vi "run.vi"(8 "error in (no error)":errorcluster, 11 "DL090202ScanHead in":refnum<class "ScanHeadDL090202.lvclass">) -> (0 "error out":errorcluster, 3 "DL090202ScanHead out":refnum<class "ScanHeadDL090202.lvclass">)   [LabVIEW 2010, in "ScanHeadDL090202.lvclass"]
uses:
  ScanHeadDL090202.lvclass
  main/labview_source/controls/undock_button.ctl
  internal_trigger_enum.ctl
  ScanHeadDL090202.lvclass/ScanHeadDL090202.ctl
  state_enum.ctl
  state_data_cluster.ctl
  GenericScanHead/GenericScanHead/GenericScanHead.lvclass
  Trajectory/GenericTrajectory/GenericTrajectory/GenericTrajectory.lvclass
  Trajectory/TrajectoryDL091126GenericVoxel/TrajectoryDL091126GenericVoxel/TrajectoryDL091126GenericVoxel.lvclass
  <vilib>/Utility/inputDevices.llb/closeKeyboard.vi
  <vilib>/Utility/inputDevices.llb/closeMouse.vi
  common/classes/ErrorController/ErrorController/class_data.vi
  <vilib>/Utility/inputDevices.llb/keyboardAcquire.vi
  <vilib>/Utility/inputDevices.llb/mouseAcquire.vi
  common/classes/ErrorController/ErrorController/ErrorController.lvclass
panel:
  in  "button:undock":T1
  in  "Tab Control":enum32{"user", "help", "debug", "about"}(tab)
  in  "zoom":dbl(slide)=1.0 min=1.0 max=20.0 step=0.1 scale=1.0..20.0
  in  "offset tabs":enum32{"fine", "coarse"}(tab)
  in  "x offset":dbl[unit](slide) scale format="%#_3g"
  in  "z offset":dbl[unit](slide)
  in  "y offset":dbl[unit](slide) scale format="%#_3g"
  in  "zero offset":bool
  in  "zero angles":bool
  in  "laser intensity (%)":dbl(slide)=14.5 caption="intensity (%)" min=0.001 max=100.0 step=0.1 scale=0.0..100.0
  in  "z angle":dbl[unit](slide) min=0.0 max=6.283185307179586 step=0.01745329238474369
  in  "x angle":dbl[unit](slide) caption="X amplitude" min=0.0 max=3.141592653589793 step=0.01745329238474369
  in  "misc tabs":enum32{"scanner-delay correction"}(tab)
  in  "x scanner":i32(slide) scale=-10.0..100.0
  in  "z scanner":i32(slide) scale=-10.0..100.0
  in  "y scanner":i32(slide) scale=-10.0..100.0
  in  "saveTrajectoryButton":bool
  out "state machine error":errorcluster
  in  "stop":bool
  out "statechart loop counter":i32
  out "evt lp error":errorcluster
  out "# elements in trigger queue":i32
  out "current action?":T2
  out "internal triggers":T2[](array[typedef])
  # "translation"
  # "rotation & tilting"
  # "Short-cuts\n\nLaser intensity: Mouse scroll wheel while space bar is pressed\n\nZoom: Mouse scroll wheel while Ctrl key is pressed\n\nToggling between horizontal and vertical plane imaging: press Ctrl-space"
  # "ScanHeadDL090202"
  # "Author: Dominik Langer, University of Zurich"
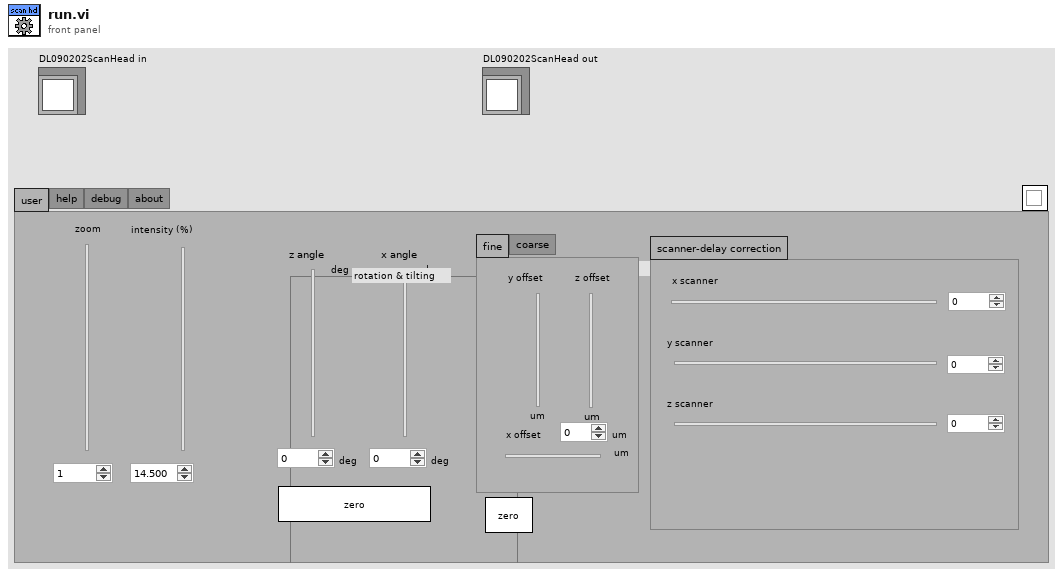
[diagram p1: front panel]
types:
  T1 = typedef "undock_button.ctl" = bool
  T2 = typedef "ScanHeadDL090202.lvclass/internal_trigger_enum.ctl" = enum16{"NULL", "initialise", "terminate", "start scanning", "stop scanning", "scale", "rotate", "tilt", "translate", "update modifiers", "fetch trajectory", "set run mode", "initialise scanners", "terminate scanners", "generate trajectory", "prepare writing", "write"}
  T3 = typedef "ScanHeadDL090202.lvclass/state_enum.ctl" = enum16{"idle", "initialising", "terminating", "writing"}
  T4 = typedef "ScanHeadDL090202.lvclass/state_data_cluster.ctl" = cluster{"already running?":bool, "new trajectory received?":bool, "fresh scan signals?":bool, "writing finished?":bool, "any trajectory received?":bool}
  T5 = enum16{"0", "1", "2", "3", "4", "5", "6", "7", "8", "9", "A", "B", "C", "D", "E", "F", "G", "H", "I", "J", "K", "L", "M", "N", "O", "P", "Q", "R", "S", "T", "U", "V", "W", "X", "Y", "Z", "F1", "F2", "F3", "F4", "F5", "F6", "F7", "F8", "F9", "F10", "F11", "F12", "F13", "F14", "F15", "ADD", "BACK", "BACKSLASH", "CAPITAL", "COMMA", "DECIMAL", "DELETE", "DIVIDE", "DOWN", "END", "EQUALS", "ESCAPE", "GRAVE (`)", "HOME", "INSERT", "LBRACKET", "LCONTROL", "LEFT", "L ALT", "LSHIFT", "LWIN", "MINUS", "MULTIPLY", "NEXT", "NUMLOCK", "NUMPAD_0", "NUMPAD_1", "NUMPAD_2", "NUMPAD_3", "NUMPAD_4", "NUMPAD_5", "NUMPAD_6", "NUMPAD_7", "NUMPAD_8", "NUMPAD_9", "PAUSE", "PERIOD", "PRIOR (PG UP)", "RBRACKET", "RCONTROL", "RETURN", "RIGHT", "R ALT", "RSHIFT", "RWIN", "SCROLL", "SEMICOLON", "SLASH", "SPACE", "SUBTRACT", "TAB", "UP", "ENTER (num pad)", "' (quote)"}
  T6 = typedef "main_trigger_enum.ctl" = enum16{"NULL", "initialise", "terminate", "start", "stop", "change objective", "change experimentController", "change imagingMode", "save notebook", "started saving", "finished saving", "expCtr ready", "expCtr missing", "imgMd ready", "imgMd missing", "scanHd ready", "scanHd missing", "DAQ ready", "DAQ missing", "imgAsm ready", "imgAsm missing", "dataColl ready", "dataColl missing", "display ready", "display missing", "analysr ready", "analysr missing", "instrmnt ready", "instrmnt missing", "stimltr ready", "stimltr missing", "stage ready", "stage missing"}
  T7 = enum16{"0", "1", "2", "3", "4", "5", "6", "7", "8", "9", "A", "B", "C", "D", "E", "F", "G", "H", "I", "J", "K", "L", "M", "N", "O", "P", "Q", "R", "S", "T", "U", "V", "W", "X", "Y", "Z", "F1", "F2", "F3", "F4", "F5", "F6", "F7", "F8", "F9", "F10", "F11", "F12", "F13", "F14", "F15", "ADD", "BACK", "BACKSLASH", "CAPITAL", "COMMA", "DECIMAL", "DELETE", "DIVIDE", "DOWN", "END", "EQUALS", "ESCAPE", "GRAVE (`)", "HOME", "INSERT", "LBRACKET", "LCONTROL", "LEFT", "L ALT", "LSHIFT", "LWIN", "MINUS", "MULTIPLY", "NEXT", "NUMLOCK", "NUMPAD_0", "NUMPAD_1", "NUMPAD_2", "NUMPAD_3", "NUMPAD_4", "NUMPAD_5", "NUMPAD_6", "NUMPAD_7", "NUMPAD_8", "NUMPAD_9", "PAUSE", "PERIOD", "PRIOR (PG UP)", "RBRACKET", "RCONTROL", "RETURN", "RIGHT", "R ALT", "RSHIFT", "RWIN", "SCROLL", "SEMICOLON", "SLASH", "SPACE", "SUBTRACT", "TAB", "UP", "ENTER (num pad)", "' (quote)"}[]
  T8 = cluster{"Horizontal":i32, "Vertical":i32, "Scrolling":i32}
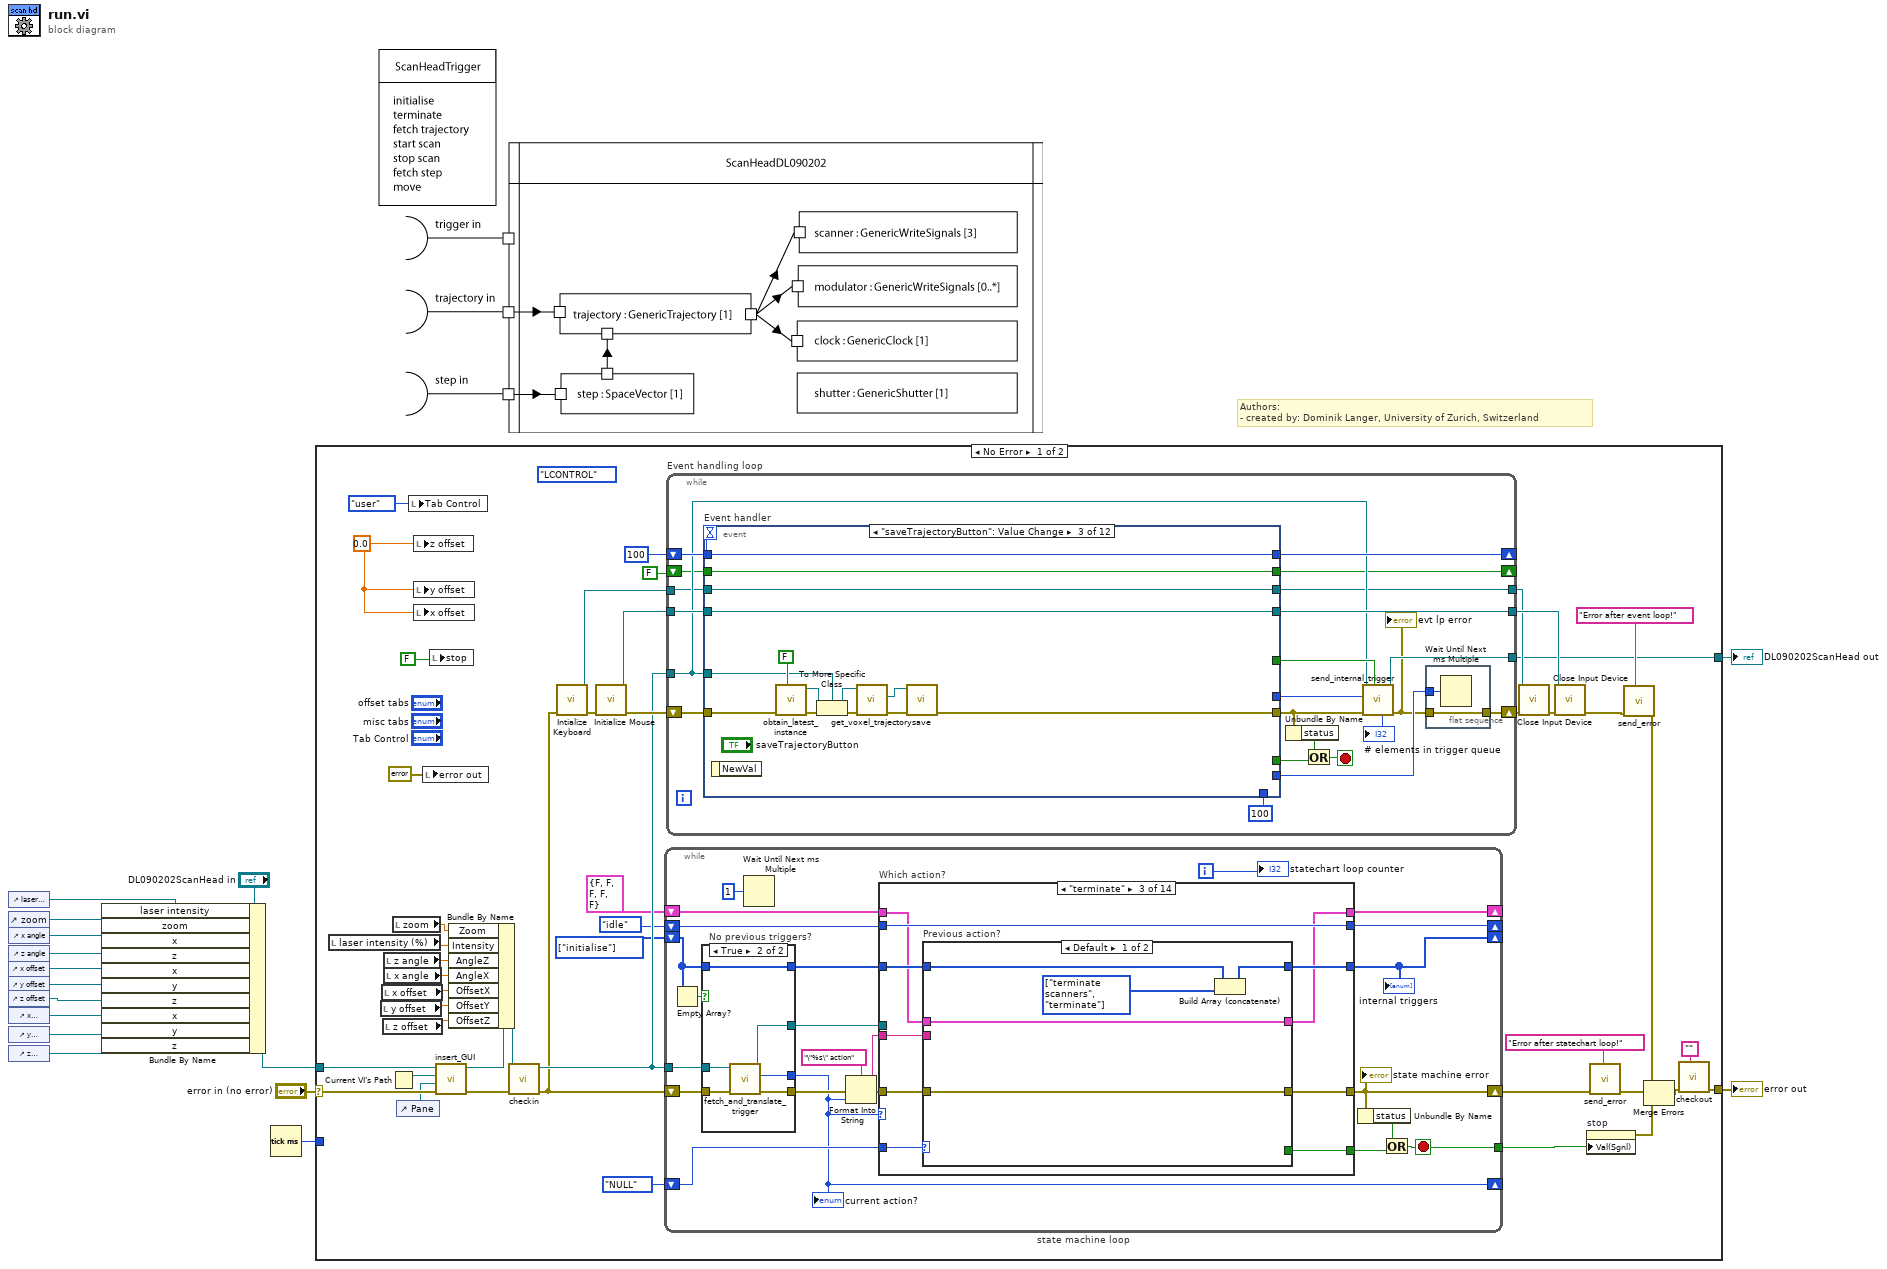
[diagram p0: block diagram]
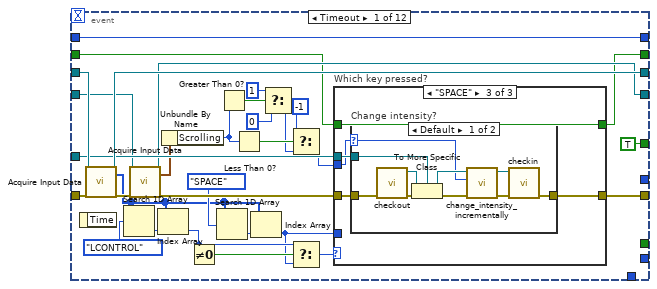
[diagram p2: hidden frame]
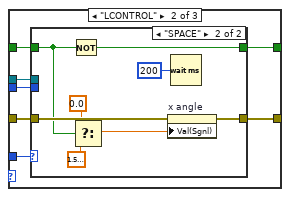
[diagram p4: hidden frame]
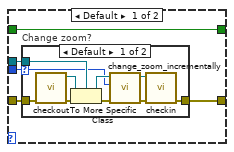
[diagram p5: hidden frame]
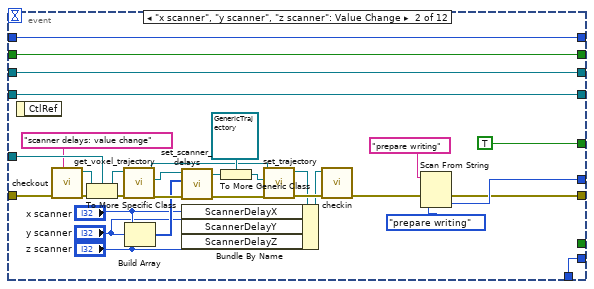
[diagram p8: hidden frame]
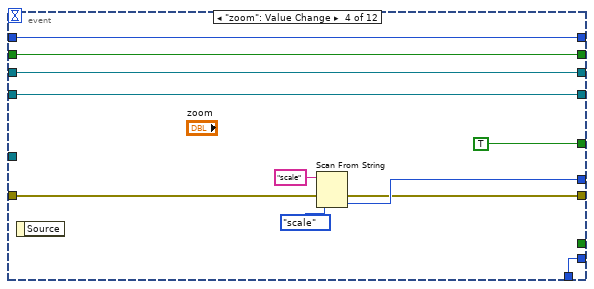
[diagram p9: hidden frame]
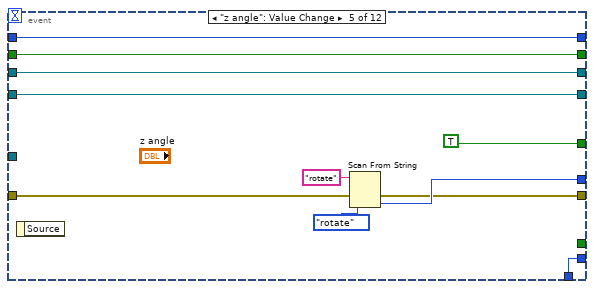
[diagram p10: hidden frame]
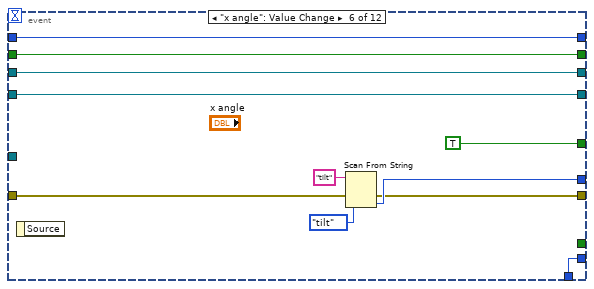
[diagram p11: hidden frame]
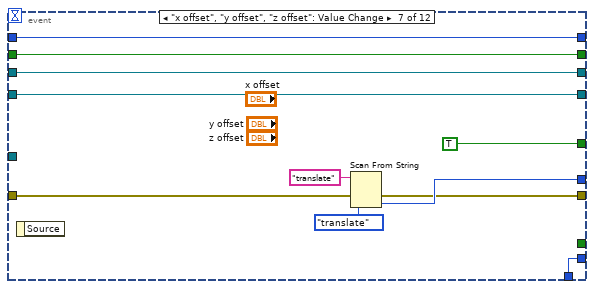
[diagram p12: hidden frame]
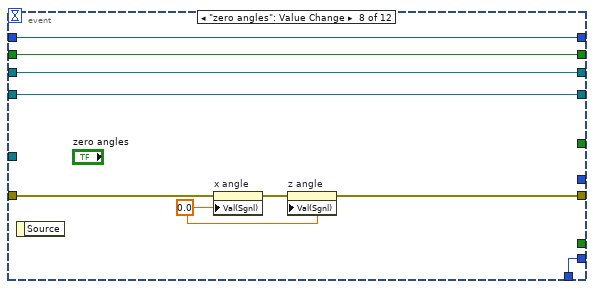
[diagram p13: hidden frame]
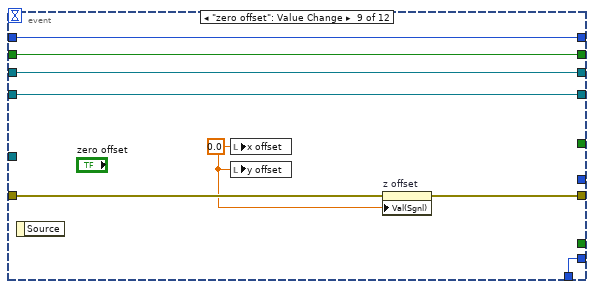
[diagram p14: hidden frame]
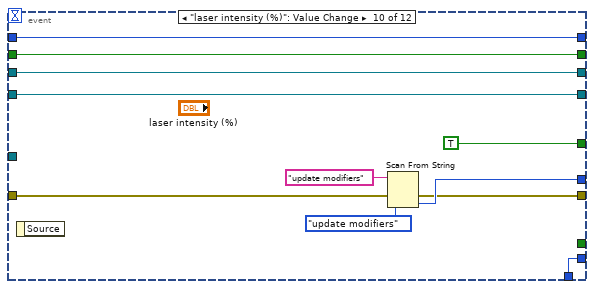
[diagram p15: hidden frame]
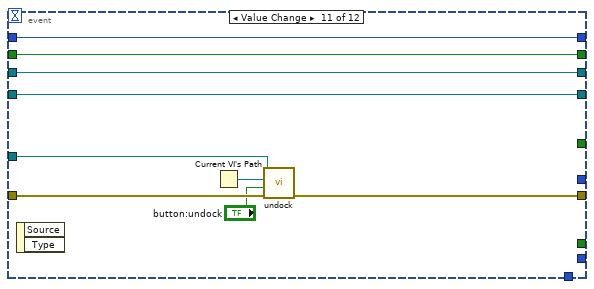
[diagram p16: hidden frame]
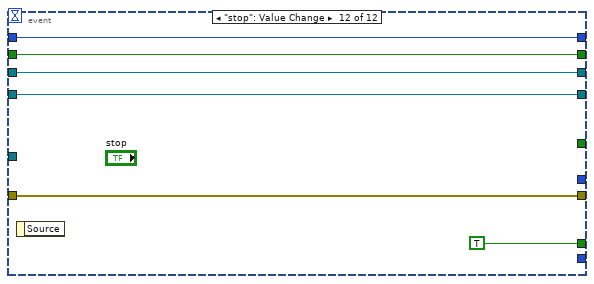
[diagram p17: hidden frame]
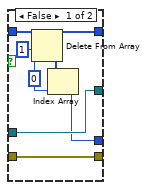
[diagram p18: hidden frame]
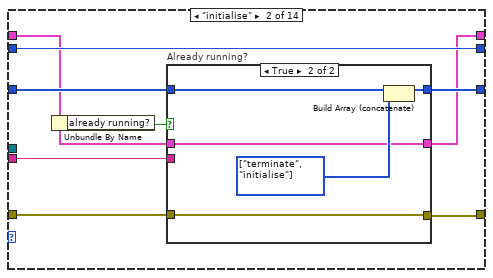
[diagram p20: hidden frame]
diagram:
  # "Authors: \n- created by: Dominik Langer, University of Zurich, Switzerland"
  n1 = control-ref of="laser intensity (%)"() -> (w9:refnum<vi>)
  n2 = control-ref of="zoom"() -> (w12:refnum<vi>)
  n3 = control-ref of="x angle"() -> (w10:refnum<vi>)
  n4 = control-ref of="z angle"() -> (w11:refnum<vi>)
  n5 = control-ref of="x offset"() -> (w6:refnum<vi>)
  n6 = control-ref of="y offset"() -> (w7:refnum<vi>)
  n7 = control-ref of="z offset"() -> (w8:refnum<vi>)
  n8 = control-ref of="x scanner"() -> (w3:refnum<vi>)
  n9 = control-ref of="y scanner"() -> (w4:refnum<vi>)
  n10 = control-ref of="z scanner"() -> (w2:refnum<vi>)
  n11 = Bundle By Name(cluster="DL090202ScanHead in", "laser intensity"=w9, "zoom"=w12, "x"=w10, "z"=w11, "x"=w6, "y"=w7, "z"=w8, "x"=w3, "y"=w4, "z"=w2) -> (w13:refnum<class "ScanHeadDL090202.lvclass">)
  n12 = Tick Count (ms)() -> (millisecond timer value=w1:u32)
  n13 = case shown="No Error" "error in (no error)" {
    selector: "error in (no error)" -> [w45 w583]
    tunnel: [w60 w583] -> w5
    tunnel: [w17 w582] -> w15
    tunnel: w13 -> [w44 w582]
    tunnel: w1 -> [_ _]
    frame No Error {
      (unwired) T5."LCONTROL" ("element")
      w25 = T2[] [enum."initialise"] items=["NULL", "initialise", "terminate", "start scanning", "stop scanning", "scale", "rotate", "tilt", "translate", "update modifiers", "fetch trajectory", "set run mode", "initialise scanners", "terminate scanners", "generate trajectory", "prepare writing", "write"]
      w55 = dbl[unit] 0.0 ("z offset")
      n14 = local read "laser intensity (%)"() -> (w52:dbl)
      n15 = local read "y offset"() -> (w47:dbl[unit])
      n16 = local read "x offset"() -> (w48:dbl[unit])
      n17 = local read "z offset"() -> (w46:dbl[unit])
      n18 = local read "z angle"() -> (w50:dbl[unit])
      n19 = local read "x angle"() -> (w49:dbl[unit])
      n20 = Current VI's Path() -> (path=w43:path)
      n21 = local read "zoom"() -> (w53:dbl)
      n22 = control-ref of="Pane"() -> (w42:refnum<vi>)
      n23 = local write "Tab Control"(enum32{"user", "help", "debug", "about"}."user" ("Tab Control")) -> ()
      n24 = local write "z offset"(w55) -> ()
      n25 = local write "y offset"(w55) -> ()
      n26 = local write "x offset"(w55) -> ()
      n27 = local write "error out"(errorcluster {"status"=FALSE, "code"=0, "source"=""} ("error out")) -> ()
      n28 = local write "stop"(FALSE) -> ()
      n29 = call-dynamic "insert_GUI.vi"("error in (no error)"=w45, "Pane"=w42, "VI path"=w43, "GenericComponent in"=w44) -> ("error out"=w28:errorcluster, "GenericComponent out"=w27:refnum<class "ScanHeadDL090202.lvclass">)  [unwired: 6 in]
      n30 = Bundle By Name(cluster=w27, "Zoom"=w53, "Intensity"=w52, "AngleZ"=w50, "AngleX"=w49, "OffsetX"=w48, "OffsetY"=w47, "OffsetZ"=w46) -> (w51:refnum<class "ScanHeadDL090202.lvclass">)
      n31 = call-dynamic "checkin.vi"("error in (no error)"=w28, "GenericScanHead in"=w51) -> ("error out"=w35:errorcluster, "GenericScanHead out"=w37:refnum<class "ScanHeadDL090202.lvclass">)  [unwired: 8 in]
      n32 = call <vilib>:"Intialize Keyboard.vi"("error in (no error)"=w35) -> ("error out"=w34:errorcluster, "device ID"=w33:refnum<k1>)  [unwired: 9 in]
      n33 = call <vilib>:"Initialize Mouse.vi"("error in (no error)"=w34) -> ("error out"=w54:errorcluster, "device ID"=w59:refnum<k1>)  [unwired: 9 in]
      n34 = while "state machine loop" {
        shift-right: [w306] -> _
        shift-left: T4 {"already running?"=FALSE, "new trajectory received?"=FALSE, "fresh scan signals?"=FALSE, "writing finished?"=FALSE, "any trajectory received?"=FALSE} -> [w307]
        tunnel: w37 -> [w321]
        shift-right: [w317] -> w23
        shift-left: w35 -> [w320]
        tunnel: [w319] -> w29
        shift-right: [w313] -> _
        shift-left: state_enum."idle" ("state") -> [w314]
        shift-right: [w312] -> _
        shift-left: w25 -> [w303]
        shift-right: [w300] -> _
        shift-left: internal_trigger_enum."NULL" ("internal trigger") -> [w305]
        i -> [w322]
        stop <- w319 stop-if-true
        n35 = Empty Array?(array=w303) -> (empty?=w304:bool)
        n36 = case "No previous triggers?" shown="True" w304 {
          tunnel: w321 -> [w328 w336]
          tunnel: w320 -> [w330 w335]
          tunnel: [w328 w334] -> w318
          tunnel: [w330 w333] -> w311
          tunnel: [w324 w332] -> w300
          tunnel: w303 -> [w329 w331]
          tunnel: [w327 w331] -> w302
          frame False {
            w325 = 0 ("index")
            n37 = Delete From Array(array=w329, length=1, index=w325) -> (deleted portion=w326:T2[], array with subset deleted=w327:T2[])
            n38 = Index Array(array=w326, index=w325) -> (element=w324:T2)
          }
          frame True {
            n39 = call-dynamic "fetch_and_translate_trigger.vi"("error in (no error)"=w335, "ScanHeadDL090202 in"=w336) -> ("error out"=w333:errorcluster, "internal trigger"=w332:T2, "ScanHeadDL090202 out"=w334:refnum<class "ScanHeadDL090202.lvclass">)  [unwired: 6 in, 1 out]
          }
        }
        "current action?" <- w300
        n40 = Wait Until Next ms Multiple(millisecond multiple=u32 1) -> ()  [unwired: 1 out]
        n41 = Format Into String(format string="\"%s\" action", error in=w311, w300) -> (resulting string=w308:string, error out=w310:errorcluster)  [unwired: 1 in]
        n42 = case "Which action?" shown="\"terminate\"" w300 {
          tunnel: w318 -> [_ _ _ w398 w412 _ _ _ w459 w474 w484 w518 w532 w553]
          tunnel: w310 -> [w338 w347 w376 w397 w411 w421 w432 w440 w453 w471 w486 w513 w530 w551]
          tunnel: [w338 w346 w375 w396 w410 w421 w432 w439 w454 w472 w485 w512 w529 w546] -> w317
          tunnel: [_ _ w368 _ _ _ _ _ _ _ _ _ _ _] -> w315
          tunnel: [w340 w349 w377 w407 w420 w422 w431 w446 w467 w482 w496 w522 w539 w558] -> w313
          tunnel: w314 -> [w340 w349 w377 w407 w420 w422 w431 w446 w467 w482 w496 w522 w539 w558]
          tunnel: w302 -> [w339 w345 w373 w406 w419 w425 w429 w438 w457 w470 w495 w511 w524 w545]
          tunnel: [w339 w344 w372 w406 w419 w424 w428 w437 w456 w469 w495 w510 w523 w545] -> w312
          tunnel: w308 -> [_ w348 w374 w399 w409 _ _ w441 w458 w473 w483 w517 w531 w552]
          tunnel: w307 -> [w337 w343 w370 w395 w408 w426 w430 w434 w466 w481 w494 w505 w528 w550]
          tunnel: [w337 w342 w369 w395 w408 w426 w430 w433 w466 w481 w494 w504 w527 w549] -> w306
          tunnel: w305 -> [_ _ w371 _ _ _ _ _ _ _ _ _ _ _]
          frame "NULL", Default {
          }
          frame "initialise" {
            n43 = Unbundle By Name(w343) -> ("already running?"=w341:bool)
            n44 = case "Already running?" shown="True" w341 {
              tunnel: w348 -> [w359 _]
              tunnel: w347 -> [w358 w367]
              tunnel: [w354 w367] -> w346
              tunnel: w345 -> [w353 w365]
              tunnel: [w353 w364] -> w344
              tunnel: w343 -> [w352 w363]
              tunnel: [w351 w363] -> w342
              frame False {
                n45 = call "checkout.vi"("locked by?"=w359, "error in (no error)"=w358) -> ("error out"=w357:errorcluster, "GenericScanHead out"=w360:refnum<class "GenericScanHead.lvclass">)  [unwired: 8 out]
                n46 = call-dynamic "construct.vi"("error in (no error)"=w357, "GenericPlugin in"=w360) -> ("error out"=w356:errorcluster, "GenericPlugin out"=w361:refnum<class "GenericScanHead.lvclass">)  [unwired: 2 in, 6 out]
                n47 = call-dynamic "initialise.vi"("error in (no error)"=w356, "GenericPlugin in"=w361) -> ("error out"=w355:errorcluster, "GenericPlugin out"=w362:refnum<class "GenericScanHead.lvclass">)  [unwired: 8 out]
                n48 = Bundle By Name(cluster=w352, "already running?"=TRUE) -> (w351:T4)
                n49 = call-dynamic "checkin.vi"("error in (no error)"=w355, "GenericScanHead in"=w362) -> ("error out"=w354:errorcluster)  [unwired: 8 in, 1 out]
              }
              frame True {
                w366 = T2[] [enum."terminate", enum."initialise"] items=["NULL", "initialise", "terminate", "start scanning", "stop scanning", "scale", "rotate", "tilt", "translate", "update modifiers", "fetch trajectory", "set run mode", "initialise scanners", "terminate scanners", "generate trajectory", "prepare writing", "write"]
                n50 = Build Array (concatenate)(w365, w366) -> (w364:T2[])
              }
            }
          }
          frame "terminate" {
            n51 = case "Previous action?" shown="Default" w371 {
              tunnel: w376 -> [w381 w390]
              tunnel: [w381 w389] -> w375
              tunnel: w374 -> [_ w388]
              tunnel: w373 -> [w379 w387]
              tunnel: [w382 w387] -> w372
              tunnel: [w380 w386] -> w369
              tunnel: w370 -> [w380 w385]
              tunnel: [_ TRUE] -> w368
              frame Default {
                w378 = T2[] [enum."terminate scanners", enum."terminate"] items=["NULL", "initialise", "terminate", "start scanning", "stop scanning", "scale", "rotate", "tilt", "translate", "update modifiers", "fetch trajectory", "set run mode", "initialise scanners", "terminate scanners", "generate trajectory", "prepare writing", "write"] ("array")
                n52 = Build Array (concatenate)(w379, w378) -> (w382:T2[])
              }
              frame "terminate scanners" {
                n53 = call "checkout.vi"("locked by?"=w388, "error in (no error)"=w390) -> ("error out"=w392:errorcluster, "GenericScanHead out"=w391:refnum<class "GenericScanHead.lvclass">)  [unwired: 8 out]
                n54 = call-dynamic "terminate.vi"("error in (no error)"=w392, "GenericPlugin in"=w391) -> ("error out"=w393:errorcluster, "GenericPlugin out"=w394:refnum<class "GenericScanHead.lvclass">)  [unwired: 8 out]
                n55 = Bundle By Name(cluster=w385, "already running?"=FALSE) -> (w386:T4)
                n56 = call-dynamic "checkin.vi"("error in (no error)"=w393, "GenericScanHead in"=w394) -> ("error out"=w389:errorcluster)  [unwired: 8 in, 1 out]
              }
            }
          }
          frame "start scanning" {
            n57 = call "checkout.vi"("locked by?"=w399, "error in (no error)"=w397) -> ("error out"=w405:errorcluster, "GenericScanHead out"=w404:refnum<class "GenericScanHead.lvclass">)  [unwired: 8 out]
            n58 = To More Specific Class(target class=w398, reference=w404, error in=w405) -> (specific class reference=w402:refnum<class "ScanHeadDL090202.lvclass">, error out=w403:errorcluster)
            n59 = call-dynamic "start.vi"("error in (no error)"=w403, "DL090202ScanHead in"=w402) -> ("error out"=w401:errorcluster, "DL090202ScanHead out"=w400:refnum<class "ScanHeadDL090202.lvclass">)  [unwired: 8 out]
            n60 = call-dynamic "checkin.vi"("error in (no error)"=w401, "GenericScanHead in"=w400) -> ("error out"=w396:errorcluster)  [unwired: 8 in, 1 out]
          }
          frame "stop scanning" {
            n61 = call "checkout.vi"("locked by?"=w409, "error in (no error)"=w411) -> ("error out"=w413:errorcluster, "GenericScanHead out"=w414:refnum<class "GenericScanHead.lvclass">)  [unwired: 8 out]
            n62 = To More Specific Class(target class=w412, reference=w414, error in=w413) -> (specific class reference=w416:refnum<class "ScanHeadDL090202.lvclass">, error out=w415:errorcluster)
            n63 = call-dynamic "stop.vi"("error in (no error)"=w415, "DL090202ScanHead in"=w416) -> ("error out"=w417:errorcluster, "DL090202ScanHead out"=w418:refnum<class "ScanHeadDL090202.lvclass">)  [unwired: 8 out]
            n64 = call-dynamic "checkin.vi"("error in (no error)"=w417, "GenericScanHead in"=w418) -> ("error out"=w410:errorcluster)  [unwired: 8 in, 1 out]
          }
          frame "scale".."tilt" {
            n65 = Build Array (concatenate)(w425, internal_trigger_enum."prepare writing" ("trigger")) -> (w424:T2[])
          }
          frame "translate", "update modifiers" {
            n66 = Build Array (concatenate)(w429, internal_trigger_enum."prepare writing" ("trigger")) -> (w428:T2[])
          }
          frame "fetch trajectory" {
            w435 = TRUE ("new trajectory received?")
            n67 = Unbundle By Name(w434) -> ("any trajectory received?"=w436:bool)
            n68 = call "checkout.vi"("locked by?"=w441, "error in (no error)"=w440) -> ("error out"=w442:errorcluster, "GenericScanHead out"=w443:refnum<class "GenericScanHead.lvclass">)  [unwired: 8 out]
            n69 = call-dynamic "fetch_trajectory.vi"("error in (no error)"=w442, "GenericScanHead in"=w443) -> ("error out"=w444:errorcluster, "GenericScanHead out"=w445:refnum<class "GenericScanHead.lvclass">)  [unwired: 8 out]
            n70 = call-dynamic "checkin.vi"("error in (no error)"=w444, "GenericScanHead in"=w445) -> ("error out"=w439:errorcluster)  [unwired: 8 in, 1 out]
            n71 = case "Any trajectory received?" shown="True" w436 {
              tunnel: w438 -> [w449 w451]
              tunnel: [w447 w450] -> w437
              frame False {
                n72 = Build Array (concatenate)(w449, internal_trigger_enum."generate trajectory" ("trigger")) -> (w447:T2[])
              }
              frame True {
                w452 = T2[] [enum."terminate scanners", enum."generate trajectory"] items=["NULL", "initialise", "terminate", "start scanning", "stop scanning", "scale", "rotate", "tilt", "translate", "update modifiers", "fetch trajectory", "set run mode", "initialise scanners", "terminate scanners", "generate trajectory", "prepare writing", "write"]
                n73 = Build Array (concatenate)(w451, w452) -> (w450:T2[])
              }
            }
            n74 = Bundle By Name(cluster=w434, "new trajectory received?"=w435, "any trajectory received?"=w435) -> (w433:T4)
          }
          frame "set run mode" {
            n75 = call "checkout.vi"("locked by?"=w458, "error in (no error)"=w453) -> ("error out"=w462:errorcluster, "GenericScanHead out"=w463:refnum<class "GenericScanHead.lvclass">)  [unwired: 8 out]
            n76 = To More Specific Class(target class=w459, reference=w463, error in=w462) -> (specific class reference=w464:refnum<class "ScanHeadDL090202.lvclass">, error out=w461:errorcluster)
            n77 = call-dynamic "update_run_mode.vi"("error in (no error)"=w461, "DL090202ScanHead in"=w464) -> ("error out"=w460:errorcluster, "DL090202ScanHead out"=w465:refnum<class "ScanHeadDL090202.lvclass">)  [unwired: 8 out]
            n78 = call-dynamic "checkin.vi"("error in (no error)"=w460, "GenericScanHead in"=w465) -> ("error out"=w454:errorcluster)  [unwired: 8 in, 1 out]
            n79 = Build Array (concatenate)(w457, internal_trigger_enum."prepare writing" ("trigger")) -> (w456:T2[])
          }
          frame "initialise scanners" {
            n80 = call "checkout.vi"("locked by?"=w473, "error in (no error)"=w471) -> ("error out"=w476:errorcluster, "GenericScanHead out"=w475:refnum<class "GenericScanHead.lvclass">)  [unwired: 8 out]
            n81 = To More Specific Class(target class=w474, reference=w475, error in=w476) -> (specific class reference=w478:refnum<class "ScanHeadDL090202.lvclass">, error out=w477:errorcluster)
            n82 = call-dynamic "initialise_scanners.vi"("error in (no error)"=w477, "DL090202ScanHead in"=w478) -> ("error out"=w479:errorcluster, "DL090202ScanHead out"=w480:refnum<class "ScanHeadDL090202.lvclass">)  [unwired: 8 out]
            n83 = call-dynamic "checkin.vi"("error in (no error)"=w479, "GenericScanHead in"=w480) -> ("error out"=w472:errorcluster)  [unwired: 8 in, 1 out]
            n84 = Build Array (concatenate)(w470, internal_trigger_enum."set run mode" ("trigger")) -> (w469:T2[])
          }
          frame "terminate scanners" {
            n85 = call "checkout.vi"("locked by?"=w483, "error in (no error)"=w486) -> ("error out"=w490:errorcluster, "GenericScanHead out"=w493:refnum<class "GenericScanHead.lvclass">)  [unwired: 8 out]
            n86 = To More Specific Class(target class=w484, reference=w493, error in=w490) -> (specific class reference=w492:refnum<class "ScanHeadDL090202.lvclass">, error out=w489:errorcluster)
            n87 = call-dynamic "terminate_scanners.vi"("error in (no error)"=w489, "DL090202ScanHead in"=w492) -> ("error out"=w488:errorcluster, "DL090202ScanHead out"=w491:refnum<class "ScanHeadDL090202.lvclass">)  [unwired: 8 out]
            n88 = call-dynamic "checkin.vi"("error in (no error)"=w488, "GenericScanHead in"=w491) -> ("error out"=w487:errorcluster)  [unwired: 8 in, 1 out]
            n89 = disable-structure shown="MAIN==1" {
              disable-tunnel: w487 -> [w499 w502]
              disable-tunnel: [w501 w502] -> w485
              frame condition #0 {
                n90 = call "string_to_main_trigger.vi"("error in (no error)"=w499, "trigger string"="scanHd missing") -> ("error out"=w498:errorcluster, "main trigger"=w500:T6)  [unwired: 8 in]
                n91 = call "send_main_trigger.vi"("error in (no error)"=w498, "trigger"=w500) -> ("error out"=w501:errorcluster)  [unwired: 9 in]
              }
              frame condition #1 (active) {
              }
            }
          }
          frame "generate trajectory" {
            n92 = call "checkout.vi"("locked by?"=w517, "error in (no error)"=w513) -> ("error out"=w516:errorcluster, "GenericScanHead out"=w520:refnum<class "GenericScanHead.lvclass">)  [unwired: 8 out]
            n93 = To More Specific Class(target class=w518, reference=w520, error in=w516) -> (specific class reference=w519:refnum<class "ScanHeadDL090202.lvclass">, error out=w515:errorcluster)
            n94 = Unbundle By Name(w505) -> ("new trajectory received?"=w508:bool)
            n95 = call-dynamic "generate_trajectory.vi"("error in (no error)"=w515, "DL090202ScanHead in"=w519) -> ("error out"=w514:errorcluster, "DL090202ScanHead out"=w521:refnum<class "ScanHeadDL090202.lvclass">)  [unwired: 8 out]
            n96 = call-dynamic "checkin.vi"("error in (no error)"=w514, "GenericScanHead in"=w521) -> ("error out"=w512:errorcluster)  [unwired: 8 in, 1 out]
            n97 = Bundle By Name(cluster=w505, "fresh scan signals?"=TRUE) -> (w504:T4)
            n98 = Select(t=internal_trigger_enum."initialise scanners" ("trigger"), s=w508, f=internal_trigger_enum."set run mode" ("trigger")) -> (s? t:f=w509:T2)
            n99 = Build Array (concatenate)(w511, w509) -> (w510:T2[])
          }
          frame "prepare writing" {
            n100 = call "checkout.vi"("locked by?"=w531, "error in (no error)"=w530) -> ("error out"=w537:errorcluster, "GenericScanHead out"=w538:refnum<class "GenericScanHead.lvclass">)  [unwired: 8 out]
            n101 = To More Specific Class(target class=w532, reference=w538, error in=w537) -> (specific class reference=w533:refnum<class "ScanHeadDL090202.lvclass">, error out=w536:errorcluster)
            n102 = call-dynamic "prepare_writing.vi"("error in (no error)"=w536, "DL090202ScanHead in"=w533) -> ("error out"=w535:errorcluster, "DL090202ScanHead out"=w534:refnum<class "ScanHeadDL090202.lvclass">)  [unwired: 1 in, 7 out]
            n103 = Build Array (concatenate)(w524, internal_trigger_enum."write" ("trigger")) -> (w523:T2[])
            n104 = call-dynamic "checkin.vi"("error in (no error)"=w535, "GenericScanHead in"=w534) -> ("error out"=w529:errorcluster)  [unwired: 8 in, 1 out]
            n105 = Bundle By Name(cluster=w528, "writing finished?"=FALSE) -> (w527:T4)
          }
          frame "write" {
            n106 = call "checkout.vi"("locked by?"=w552, "error in (no error)"=w551) -> ("error out"=w555:errorcluster, "GenericScanHead out"=w554:refnum<class "GenericScanHead.lvclass">)  [unwired: 8 out]
            n107 = To More Specific Class(target class=w553, reference=w554, error in=w555) -> (specific class reference=w557:refnum<class "ScanHeadDL090202.lvclass">, error out=w556:errorcluster)
            n108 = call-dynamic "write_signals.vi"("error in (no error)"=w556, "DL090202ScanHead in"=w557) -> ("error out"=w548:errorcluster, "finished?"=w544:bool, "DL090202ScanHead out"=w547:refnum<class "ScanHeadDL090202.lvclass">)  [unwired: 7 out]
            n109 = case "Writing finished?" shown="False" w544 {
              selector: w544 -> [_ w572]
              tunnel: w550 -> [w568 w575]
              tunnel: [w568 w574] -> w549
              tunnel: w548 -> [w562 w571]
              tunnel: w547 -> [w567 w570]
              tunnel: ["NULL" "scanHd ready"] -> w543
              tunnel: [w566 w571] -> w541
              tunnel: [w565 w570] -> w542
              frame False {
                n110 = Scan From String(input string="write", error in=w562, default 1=internal_trigger_enum."write" ("trigger")) -> (error out=w561:errorcluster, output 1=w563:T2)  [unwired: 2 in, 2 out]
                n111 = call-dynamic "send_internal_trigger.vi"("error in (no error)"=w561, "trigger"=w563, "DL090202ScanHead in"=w567) -> ("error out"=w566:errorcluster, "DL090202ScanHead out"=w565:refnum<class "ScanHeadDL090202.lvclass">)  [unwired: 1 in, 6 out]
              }
              frame True {
                w573 = FALSE
                n112 = Bundle By Name(cluster=w575, "new trajectory received?"=w573, "fresh scan signals?"=w573, "writing finished?"=w572) -> (w574:T4)
              }
            }
            n113 = call-dynamic "checkin.vi"("error in (no error)"=w541, "GenericScanHead in"=w542) -> ("error out"=w540:errorcluster)  [unwired: 8 in, 1 out]
            n114 = disable-structure shown="MAIN==1" {
              disable-tunnel: w540 -> [w577 w581]
              disable-tunnel: [w580 w581] -> w546
              disable-tunnel: w543 -> [w579 _]
              frame condition #0 {
                n115 = call "string_to_main_trigger.vi"("error in (no error)"=w577, "trigger string"=w579) -> ("error out"=w576:errorcluster, "main trigger"=w578:T6)  [unwired: 8 in]
                n116 = call "send_main_trigger.vi"("error in (no error)"=w576, "trigger"=w578) -> ("error out"=w580:errorcluster)  [unwired: 9 in]
              }
              frame condition #1 (active) {
              }
            }
          }
        }
        "state machine error" <- w317
        "internal triggers" <- w312
        n117 = Unbundle By Name(w317) -> ("status"=w316:bool)
        n118 = Or(x=w316, y=w315) -> (x .or. y?=w319:bool)
        "statechart loop counter" <- w322
      }
      n119 = while "Event handling loop" {
        shift-right: [w82] -> _
        shift-left: 100 -> [w83]
        tunnel: w37 -> [w77]
        tunnel: [w81] -> w17
        tunnel: w59 -> [w79]
        tunnel: [w78] -> w58
        tunnel: w33 -> [w72]
        tunnel: [w71] -> w32
        shift-right: [w65] -> w31
        shift-left: w54 -> [w84]
        shift-right: [w67] -> _
        shift-left: FALSE -> [w68]
        stop <- w74 stop-if-true
        n120 = event "Event handler" shown="[2] \"saveTrajectoryButton\": Value Change" {
          selector: _ -> [_ _ _ _ _ _ _ _ _ _ _ _]
          dyn-events: _ -> [_ _ _ _ _ _ _ _ _ _ _ _]
          timeout: w83 -> [_ _ _ _ _ _ _ _ _ _ _ _]
          tunnel: w84 -> [w115 w194 w209 w216 w226 w238 w248 w264 w272 w277 w289 w299]
          tunnel: [w111 w170 w201 w215 w227 w237 w249 w262 w271 w276 w288 w299] -> w76
          tunnel: [w117 w198 w212 w223 w234 w245 w256 w265 w273 w284 w293 w298] -> w82
          tunnel: w83 -> [w117 w198 w212 w223 w234 w245 w256 w265 w273 w284 w293 w298]
          tunnel: [_ _ _ _ _ _ _ _ _ _ _ TRUE] -> w73
          tunnel: [TRUE TRUE _ TRUE TRUE TRUE TRUE _ _ TRUE _ _] -> w80
          tunnel: w77 -> [w110 w195 w208 _ _ _ _ _ _ _ w290 _]
          tunnel: [_ w173 _ w217 w228 w239 w250 _ _ w279 _ _] -> w69
          tunnel: w79 -> [w106 w197 w211 w221 w232 w243 w254 w260 w269 w282 w292 w296]
          tunnel: [w105 w197 w211 w221 w232 w243 w254 w260 w269 w282 w292 w296] -> w78
          tunnel: w72 -> [w116 w169 w200 w220 w231 w242 w253 w259 w268 w281 w291 w295]
          tunnel: [w113 w169 w200 w220 w231 w242 w253 w259 w268 w281 w291 w295] -> w71
          tunnel: w68 -> [w88 w168 w199 w214 w225 w236 w247 w258 w267 w275 w285 w294]
          tunnel: [w87 w168 w199 w214 w225 w236 w247 w258 w267 w275 w285 w294] -> w67
          tunnel: [_ w167 _ w213 w224 w235 w246 w257 w266 w274 _ _] -> w66
          tunnel: u32 100 ("millisecond multiple") -> [_ w167 _ w213 w224 w235 w246 w257 w266 w274 _ _]
          event Timeout {
            n121 = event-data() -> ()  [unwired: 2 out]
            n122 = call-poly <vilib>:"Acquire Input Data.vi"("device ID"=w116, "error in (no error)"=w115) -> ("device ID"=w113:refnum<k1>, "keys pressed"=w102:T7, "error out"=w108:errorcluster)  [unwired: 15 in]
            n123 = Search 1D Array(1D array=w102, element=T5."LCONTROL") -> (index of element=w109:i32)  [unwired: 1 in]
            n124 = call-poly <vilib>:"Acquire Input Data.vi"("device ID"=w106, "error in (no error)"=w108) -> ("device ID"=w105:refnum<k1>, "axis info"=w104:T8, "error out"=w107:errorcluster)  [unwired: 14 in, 1 out]
            n125 = Index Array(array=w102, index=w109) -> (element=w100:T5)
            n126 = Unbundle By Name(w104) -> ("Scrolling"=w92:i32)
            n127 = Not Equal To 0?(x=w100) -> (x != 0?=w99:bool)
            n128 = Search 1D Array(1D array=w102, element=T5."SPACE") -> (index of element=w101:i32)  [unwired: 1 in]
            n129 = Greater Than 0?(x=w92) -> (x > 0?=w97:bool)
            n130 = Less Than 0?(x=w92) -> (x < 0?=w95:bool)
            n131 = Index Array(array=w102, index=w101) -> (element=w89:T5)
            n132 = Select(t=1, s=w97, f=0) -> (s? t:f=w93:i32)
            n133 = Select(t=-1, s=w95, f=w93) -> (s? t:f=w91:i32)
            n134 = Select(t=w100, s=w99, f=w89) -> (s? t:f=w98:T5)
            n135 = case "Which key pressed?" shown="\"SPACE\"" w98 {
              tunnel: w107 -> [w119 w125 w154]
              tunnel: [w119 w126 w153] -> w111
              tunnel: w110 -> [_ w124 w155]
              tunnel: w91 -> [_ w123 w152]
              tunnel: w89 -> [_ w122 _]
              tunnel: w88 -> [w118 w121 w151]
              tunnel: [w118 w120 w151] -> w87
              frame Default {
              }
              frame "LCONTROL" {
                n136 = case shown="\"SPACE\"" w122 {
                  tunnel: [w131 w149] -> w126
                  tunnel: w125 -> [w130 w150]
                  tunnel: w124 -> [w129 _]
                  tunnel: w123 -> [w128 _]
                  tunnel: w121 -> [w127 w144]
                  tunnel: [w127 w148] -> w120
                  frame Default {
                    n137 = case "Change zoom?" shown="Default" w128 {
                      selector: w128 -> [w132 _]
                      tunnel: w130 -> [w138 w142]
                      tunnel: [w140 w142] -> w131
                      tunnel: w129 -> [w134 _]
                      frame Default {
                        n138 = call "checkout.vi"("error in (no error)"=w138) -> ("error out"=w137:errorcluster, "GenericScanHead out"=w135:refnum<class "GenericScanHead.lvclass">)  [unwired: 9 in]
                        n139 = To More Specific Class(target class=w134, reference=w135, error in=w137) -> (specific class reference=w133:refnum<class "ScanHeadDL090202.lvclass">, error out=w136:errorcluster)
                        n140 = call "change_zoom_incrementally.vi"("error in (no error)"=w136, "mode"=w132, "ScanHeadDL090202 in"=w133) -> ("error out"=w141:errorcluster, "ScanHeadDL090202 out"=w139:refnum<class "ScanHeadDL090202.lvclass">)  [unwired: 7 in]
                        n141 = call-dynamic "checkin.vi"("error in (no error)"=w141, "GenericScanHead in"=w139) -> ("error out"=w140:errorcluster)  [unwired: 8 in, 1 out]
                      }
                      frame 0 {
                      }
                    }
                  }
                  frame "SPACE" {
                    n142 = Not(x=w144) -> (.not. x?=w148:bool)
                    n143 = Select(t=dbl[unit] 0.0 ("Value (Signaling)"), s=w144, f=dbl[unit] 1.5707963267948966) -> (s? t:f=w146:dbl[unit])
                    n144 = property on="x angle" class="Slide (strict)"(error in=w150, "Val(Sgnl)"=w146) -> (error out=w149:errorcluster)  [unwired: 1 in, 1 out]
                    n145 = Wait (ms)(milliseconds to wait=u32 200) -> ()  [unwired: 1 out]
                  }
                }
              }
              frame "SPACE" {
                n146 = case "Change intensity?" shown="Default" w152 {
                  selector: w152 -> [w156 _]
                  tunnel: w154 -> [w164 w166]
                  tunnel: [w165 w166] -> w153
                  tunnel: w155 -> [w161 _]
                  frame Default {
                    n147 = call "checkout.vi"("error in (no error)"=w164) -> ("error out"=w163:errorcluster, "GenericScanHead out"=w162:refnum<class "GenericScanHead.lvclass">)  [unwired: 9 in]
                    n148 = To More Specific Class(target class=w161, reference=w162, error in=w163) -> (specific class reference=w157:refnum<class "ScanHeadDL090202.lvclass">, error out=w160:errorcluster)
                    n149 = call "change_intensity_incrementally.vi"("error in (no error)"=w160, "mode"=w156, "ScanHeadDL090202 in"=w157) -> ("error out"=w159:errorcluster, "ScanHeadDL090202 out"=w158:refnum<class "ScanHeadDL090202.lvclass">)  [unwired: 7 in]
                    n150 = call-dynamic "checkin.vi"("error in (no error)"=w159, "GenericScanHead in"=w158) -> ("error out"=w165:errorcluster)  [unwired: 8 in, 1 out]
                  }
                  frame 0 {
                  }
                }
              }
            }
          }
          event "x scanner", "y scanner", "z scanner": Value Change {
            n151 = event-data() -> ()  [unwired: 2 out]
            n152 = call "checkout.vi"("locked by?"="scanner delays: value change", "error in (no error)"=w194) -> ("error out"=w196:errorcluster, "GenericScanHead out"=w181:refnum<class "GenericScanHead.lvclass">)  [unwired: 8 in]
            n153 = To More Specific Class(target class=w195, reference=w181, error in=w196) -> (specific class reference=w192:refnum<class "ScanHeadDL090202.lvclass">, error out=w183:errorcluster)
            n154 = call-dynamic "get_voxel_trajectory.vi"("error in (no error)"=w183, "ScanHeadDL090202 in"=w192) -> ("error out"=w191:errorcluster, "trajectory"=w190:refnum<class "TrajectoryDL091126GenericVoxel.lvclass">, "ScanHeadDL090202 out"=w184:refnum<class "ScanHeadDL090202.lvclass">)  [unwired: 7 in]
            n155 = Build Array("x scanner", "y scanner", "z scanner") -> (w182:i32[])
            n156 = call-dynamic "set_scanner_delays.vi"("error in (no error)"=w191, "scanner delays"=w182, "TrajectoryDL091126GenericVoxel in"=w190) -> ("error out"=w187:errorcluster, "TrajectoryDL091126GenericVoxel out"=w188:refnum<class "TrajectoryDL091126GenericVoxel.lvclass">)  [unwired: 7 in]
            n157 = To More Generic Class(target class=refnum<class "GenericTrajectory.lvclass"> refnum ("GenericTrajectory.lvclass"), reference=w188) -> (generic class reference=w186:refnum<class "GenericTrajectory.lvclass">)
            n158 = call-dynamic "set_trajectory.vi"("error in (no error)"=w187, "trajectory"=w186, "GenericScanHead.lvclass in"=w184) -> ("error out"=w185:errorcluster, "GenericScanHead.lvclass out"=w179:refnum<class "ScanHeadDL090202.lvclass">)  [unwired: 7 in]
            n159 = Bundle By Name(cluster=w179, "ScannerDelayX"="x scanner", "ScannerDelayY"="y scanner", "ScannerDelayZ"="z scanner") -> (w178:refnum<class "ScanHeadDL090202.lvclass">)
            n160 = call-dynamic "checkin.vi"("error in (no error)"=w185, "GenericScanHead in"=w178) -> ("error out"=w171:errorcluster)  [unwired: 8 in, 1 out]
            n161 = Scan From String(input string="prepare writing", error in=w171, default 1=internal_trigger_enum."prepare writing" ("trigger")) -> (error out=w170:errorcluster, output 1=w173:T2)  [unwired: 2 in, 2 out]
          }
          event "saveTrajectoryButton": Value Change {
            n162 = event-data() -> ()  [unwired: 2 out]
            n163 = call "obtain_latest_instance.vi"("quick, but maybe outdated?"=FALSE, "error in (no error)"=w209) -> ("error out"=w206:errorcluster, "GenericScanHead out"=w207:refnum<class "GenericScanHead.lvclass">)  [unwired: 8 in]
            n164 = To More Specific Class(target class=w208, reference=w207, error in=w206) -> (specific class reference=w204:refnum<class "ScanHeadDL090202.lvclass">, error out=w205:errorcluster)
            n165 = call-dynamic "get_voxel_trajectory.vi"("error in (no error)"=w205, "ScanHeadDL090202 in"=w204) -> ("error out"=w203:errorcluster, "trajectory"=w202:refnum<class "TrajectoryDL091126GenericVoxel.lvclass">)  [unwired: 7 in, 1 out]
            n166 = call-dynamic "save.vi"("error in (no error)"=w203, "TrajectoryDL091126GenericVoxel in"=w202) -> ("error out"=w201:errorcluster)  [unwired: 8 in, 1 out]
          }
          event "zoom": Value Change {
            n167 = event-data() -> ()  [unwired: 2 out]
            n168 = Scan From String(input string="scale", error in=w216, default 1=internal_trigger_enum."scale" ("trigger")) -> (error out=w215:errorcluster, output 1=w217:T2)  [unwired: 2 in, 2 out]
          }
          event "z angle": Value Change {
            n169 = event-data() -> ()  [unwired: 2 out]
            n170 = Scan From String(input string="rotate", error in=w226, default 1=internal_trigger_enum."rotate" ("trigger")) -> (error out=w227:errorcluster, output 1=w228:T2)  [unwired: 2 in, 2 out]
          }
          event "x angle": Value Change {
            n171 = event-data() -> ()  [unwired: 2 out]
            n172 = Scan From String(input string="tilt", error in=w238, default 1=internal_trigger_enum."tilt" ("trigger")) -> (error out=w237:errorcluster, output 1=w239:T2)  [unwired: 2 in, 2 out]
          }
          event "x offset", "y offset", "z offset": Value Change {
            n173 = event-data() -> ()  [unwired: 2 out]
            n174 = Scan From String(input string="translate", error in=w248, default 1=internal_trigger_enum."translate" ("trigger")) -> (error out=w249:errorcluster, output 1=w250:T2)  [unwired: 2 in, 2 out]
          }
          event "zero angles": Value Change {
            w261 = dbl[unit] 0.0 ("Value (Signaling)")
            n175 = event-data() -> ()  [unwired: 2 out]
            n176 = property on="x angle" class="Slide (strict)"(error in=w264, "Val(Sgnl)"=w261) -> (error out=w263:errorcluster)  [unwired: 1 in, 1 out]
            n177 = property on="z angle" class="Slide (strict)"(error in=w263, "Val(Sgnl)"=w261) -> (error out=w262:errorcluster)  [unwired: 1 in, 1 out]
          }
          event "zero offset": Value Change {
            w270 = dbl[unit] 0.0 ("x offset")
            n178 = event-data() -> ()  [unwired: 2 out]
            n179 = local write "x offset"(w270) -> ()
            n180 = local write "y offset"(w270) -> ()
            n181 = property on="z offset" class="Slide (strict)"(error in=w272, "Val(Sgnl)"=w270) -> (error out=w271:errorcluster)  [unwired: 1 in, 1 out]
          }
          event "laser intensity (%)": Value Change {
            n182 = event-data() -> ()  [unwired: 2 out]
            n183 = Scan From String(input string="update modifiers", error in=w277, default 1=internal_trigger_enum."update modifiers" ("trigger")) -> (error out=w276:errorcluster, output 1=w279:T2)  [unwired: 2 in, 2 out]
          }
          event Value Change {
            n184 = event-data() -> ()  [unwired: 3 out]
            n185 = Current VI's Path() -> (path=w286:path)
            n186 = call-dynamic "undock.vi"("error in (no error)"=w289, "undock?"="button:undock", "VI path"=w286, "component in"=w290) -> ("error out"=w288:errorcluster)  [unwired: 6 in, 1 out]
          }
          event "stop": Value Change {
            n187 = event-data() -> ()  [unwired: 2 out]
          }
        }
        n188 = Unbundle By Name(w76) -> ("status"=w75:bool)
        n189 = Or(x=w75, y=w73) -> (x .or. y?=w74:bool)
        n190 = call-dynamic "send_internal_trigger.vi"("ensure unique insertion?"=w80, "error in (no error)"=w76, "trigger"=w69, "DL090202ScanHead in"=w77) -> ("error out"=w64:errorcluster, "DL090202ScanHead out"=w81:refnum<class "ScanHeadDL090202.lvclass">, "# elements in queue"=→"# elements in trigger queue":i32)  [unwired: 5 out]
        "evt lp error" <- w64
        n191 = flat-sequence {
          tunnel: w66 -> [w86]
          tunnel: [w85] -> w65
          tunnel: w64 -> [w85]
          frame #0 {
            n192 = Wait Until Next ms Multiple(millisecond multiple=w86) -> ()  [unwired: 1 out]
          }
        }
      }
      n193 = call-poly <vilib>:"Close Input Device.vi"("error in (no error)"=w31, "device ID"=w32) -> ("error out"=w30:errorcluster)  [unwired: 8 in]
      n194 = call-poly <vilib>:"Close Input Device.vi"("error in (no error)"=w30, "device ID"=w58) -> ("error out"=w18:errorcluster)  [unwired: 8 in]
      n195 = property on="stop" class="Bool (strict)"("Val(Sgnl)"=w29) -> (error out=w22:errorcluster)  [unwired: 2 in, 1 out]
      n196 = call "send_error.vi"("additional message"="Error after statechart loop!", "error in (no error)"=w23) -> ("error out"=w41:errorcluster)  [unwired: 9 in]
      n197 = call "send_error.vi"("additional message"="Error after event loop!", "error in (no error)"=w18) -> ("error out"=w39:errorcluster)  [unwired: 9 in]
      n198 = Merge Errors(w39, w41, w22) -> (w57:errorcluster)
      n199 = call "checkout.vi"("locked by?"="", "error in (no error)"=w57) -> ("error out"=w60:errorcluster)  [unwired: 9 out]
    }
    frame Error {
    }
  }
  "error out" <- w5
  "DL090202ScanHead out" <- w15
